vi "+-math.vi"(9 "S":dbl format="%#_13g", 10 "VMAX":dbl format="%#_13g", 11 "ACC":dbl format="%#_13g") -> (1 "T2":dbl, 2 "T3":dbl, 3 "T1":dbl)   [LabVIEW 2018]
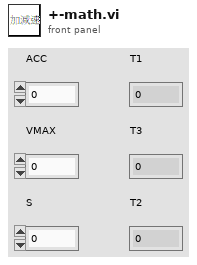
[diagram p1: front panel]
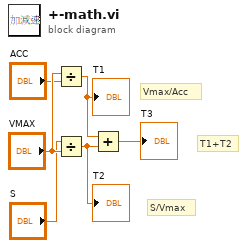
[diagram p0: block diagram]
diagram:
  # "T1+T2"
  # "S/Vmax"
  # "Vmax/Acc"
  n1 = Divide(x="VMAX", y="ACC") -> (x/y=w4:dbl)
  "T1" <- w4
  n2 = Divide(x="S", y="VMAX") -> (x/y=w5:dbl)
  "T2" <- w5
  n3 = Add(x=w4, y=w5) -> (x+y=→"T3":dbl)
